vi "Evaluate with new Params.vi"(8 "error in (no error)":errorcluster, 11 "HIJ Vision Display in":refnum<class "HIJ Vision Display.lvclass">) -> (0 "error out":errorcluster, 3 "HIJ Vision Display out":refnum<class "HIJ Vision Display.lvclass">)   [LabVIEW 2020, in "HIJ Vision Display.lvlib" / "HIJ Vision Display.lvclass"]
uses:
  HIJ Vision Display.lvclass
  HIJ Vision Display.lvclass/HIJ Vision Display.ctl
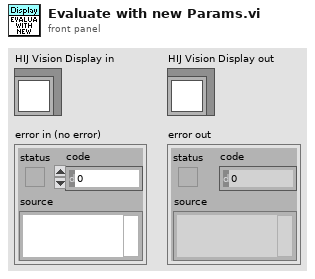
[diagram p1: front panel]
types:
  T1 = typedef "IMAQ Image.ctl" = refnum<image>
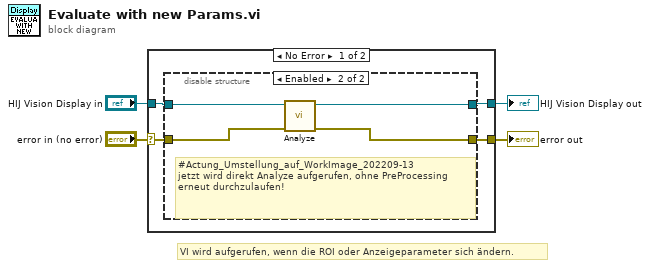
[diagram p0: block diagram]
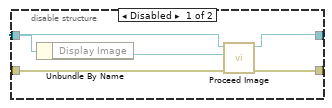
[diagram p2: hidden frame]
diagram:
  # "VI wird aufgerufen, wenn die ROI oder Anzeigeparameter sich ändern."
  n1 = case shown="No Error" "error in (no error)" {
    selector: "error in (no error)" -> [w6 w19]
    tunnel: [w5 w19] -> w3
    tunnel: [w8 w18] -> w1
    tunnel: "HIJ Vision Display in" -> [w7 w18]
    frame No Error {
      n2 = disable-structure shown="Enabled" {
        disable-tunnel: [w13 w17] -> w8
        disable-tunnel: w7 -> [w12 w16]
        disable-tunnel: w6 -> [w11 w15]
        disable-tunnel: [w10 w14] -> w5
        frame Disabled {
          n3 = Unbundle By Name(w12) -> ("Display Image"=w9:T1)
          n4 = call "Proceed Image.vi"("error in (no error)"=w11, "Image"=w9, "IMAQ Display in"=w12) -> ("error out"=w10:errorcluster, "HIJ Vision Display out"=w13:refnum<class "HIJ Vision Display.lvclass">)  [unwired: 7 in]
        }
        frame Enabled {
          # "#Actung_Umstellung_auf_WorkImage_202209-13\njetzt wird direkt Analyze aufgerufen, ohne PreProcessing\nerneut durchzulaufen!"
          n5 = call-dynamic "Analyze.vi"("error in (no error)"=w15, "HIJ Vision Display in"=w16) -> ("error out"=w14:errorcluster, "HIJ Vision Display out"=w17:refnum<class "HIJ Vision Display.lvclass">)  [unwired: 8 in]
        }
      }
    }
    frame Error {
    }
  }
  "error out" <- w3
  "HIJ Vision Display out" <- w1
